vi "DB UI - Search-Load Setup.vi"(8 "error in (no error)":errorcluster, 11 "Refnums":T4) -> (0 "Error Out":errorcluster, 1 "{Cancel}":bool, 2 "Transaction":T3, 3 "1D Results":string[](array[string]))   [LabVIEW 2020]
uses:
  Control/Combo Box.ctl
  Control/DB - Refnums.ctl
  Control/Setup - Part Details - Item Details.ctl
  <vilib>/Utility/miscctls.llb/LVRectTypeDef.ctl
  Control/Transaction Cluster.ctl
  Control/Debug Tab.ctl
  <vilib>/Utility/miscctls.llb/LVRowAndColumnUnsignedTypeDef.ctl
  <vilib>/Utility/miscctls.llb/LVPointTypeDef.ctl
  <vilib>/Utility/miscctls.llb/LVRowAndColumnTypeDef.ctl
  Control/DB - Setup Item Enum.ctl
panel:
  in  "OR [CaptionOnly]":string caption="OR"
  in  "Tab Control":T1
  out "Get Clicked Column Header":i32
  in  "Ascending":bool
  out "Time":u32
  out "x":u32
  out "y":u32
  out "Front Panel Window:Panel Bounds":T2
  out "2D Results":string[][](array[string])=[["Production", "OperationNo1"], ["Production", "Qty1"], ["Production", "NCRNo1"], ["Production", "CustomerID1"], ["Production", "Customer1"], ["Production", "Project1"], ["Production", "SalesOrderNo1"], ["Production", "SalesOrderItemNo1"], ["Production", "MaterialNo1"], ["Production", "MaterialRev1"], ["Production", "MaterialDesc1"], ["Production", "SerialNos1"], ["Production", "UnitOfQty1"]]
  out "Drop Down":bool
  in  "CellBG New Cells":u32(colorbox)=16777225
  in  "CellBG Unused Cells":u32(colorbox)=16777238
  in  "CellBG ColHdrs":u32(colorbox)=11776947
  out "MHandler Error":errorcluster
  in  "Criteria [CaptionOnly]":string caption="Criteria"
  in  "Cancel":bool caption="Report Execute Search"
  in  "Open":bool caption="Report Execute Search"
  in  "Search":bool caption="Report Execute Search"
  in  "Report List":i32(listbox)=-1 caption="List"
  in  "OrderNo":T5 caption="Order No."
  in  "TransactionNo":T5 caption="Transaction No."
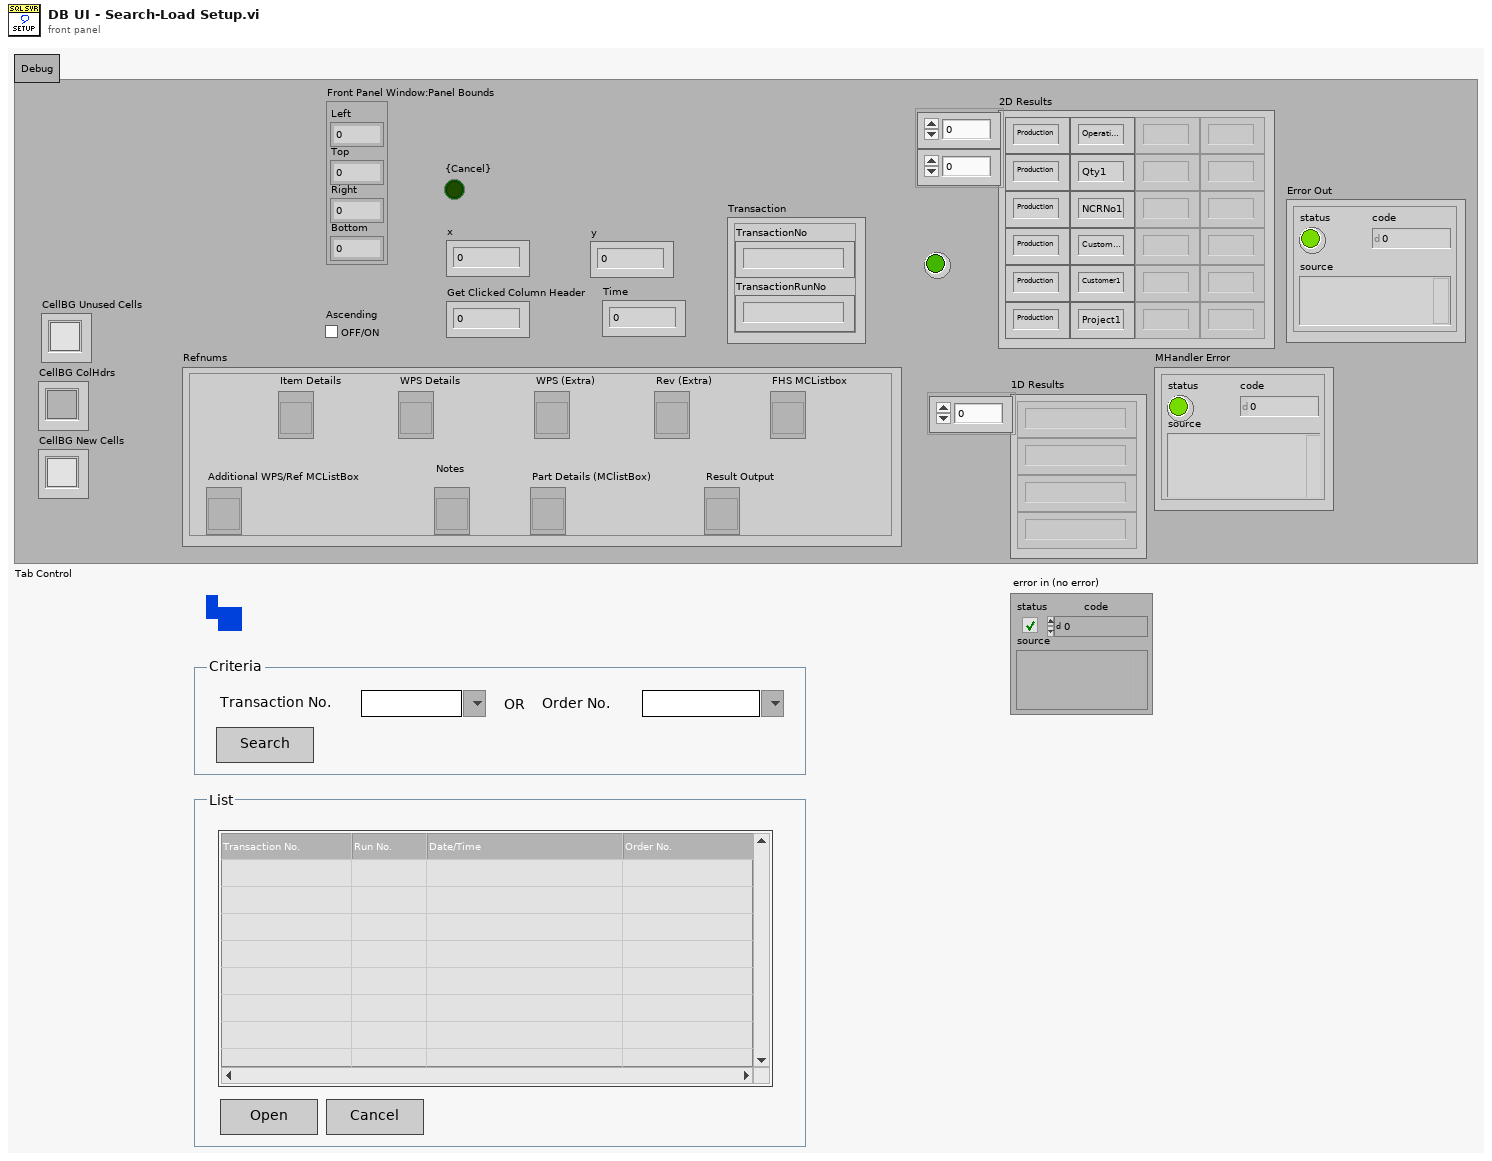
[diagram p1: front panel]
types:
  T1 = typedef "Debug Tab.ctl" = enum32{"Debug"}
  T2 = typedef "LVRectTypeDef.ctl" = cluster{"Left":i16, "Top":i16, "Right":i16, "Bottom":i16}
  T3 = typedef "Transaction Cluster.ctl" = cluster{"TransactionNo":string, "TransactionRunNo":string}
  T4 = typedef "DB - Refnums.ctl" = cluster{"Item Details":refnum<vi>, "WPS Details":refnum<vi>, "WPS (Extra)":refnum<vi>, "Rev (Extra) ":refnum<vi>, "FHS MCListbox":refnum<vi>, "Additional WPS/Ref MCListBox":refnum<vi>, "Notes":refnum<vi>, "Part Details (MClistBox)":refnum<vi>, "Result Output":refnum<vi>}
  T5 = typedef "Combo Box.ctl" = string
  T6 = typedef "LVPointTypeDef.ctl" = cluster{"Horizontal":i16, "Vertical":i16}
  T7 = typedef "LVRowAndColumnUnsignedTypeDef.ctl" = cluster{"Row":u32, "Column":u32}
  T8 = typedef "LVRowAndColumnTypeDef.ctl" = cluster{"Row":i32, "Column":i32}
  T9 = typedef "DB - Setup Item Enum.ctl" = enum16{"SELECT [Plant],[OrderNo]", "INSERT [Setup].[Header]", "INSERT [Setup].[Item]", "INSERT [Setup].[ProcedureItem]", "SELECT [TransactionNo]", "SELECT [TransactionNo], others", "SELECT [OrderNo]", "SELECT [OrderNo], others", "SELECT h.[TransactionNo], i.[OrderNo]", "SELECT [Setup].[ProcedureItem]", "SELECT [EquipmentxId]"}
  T10 = enum8{"Enabled", "Disabled", "Disabled and Grayed Out"}
  T11 = cluster{"TransactionNo":string, "TransactionRunNo":string}
  T12 = typedef "eventvkey.ctl" = enum16{"ASCII", "Enter", "Return", "Shift", "Ctrl", "Alt", "Cmd", "Opt", "Caps", "NumLock", "Clear", "Break", "Up", "Down", "Left", "Right", "Insert", "Delete", "Home", "End", "PageUp", "PageDown", "Escape", "Help", "Pause", "ScrollLock", "F1", "F2", "F3", "F4", "F5", "F6", "F7", "F8", "F9", "F10", "F11", "F12", "F13", "F14", "F15", "F16", "F17", "F18", "F19", "F20", "F21", "F22", "F23", "F24", "Play", "VolumeUp", "VolumeDown", "Mute", "Two Byte Char"}
  T13 = typedef "LVPoint32TypeDef.ctl" = cluster{"Horizontal":i32, "Vertical":i32}
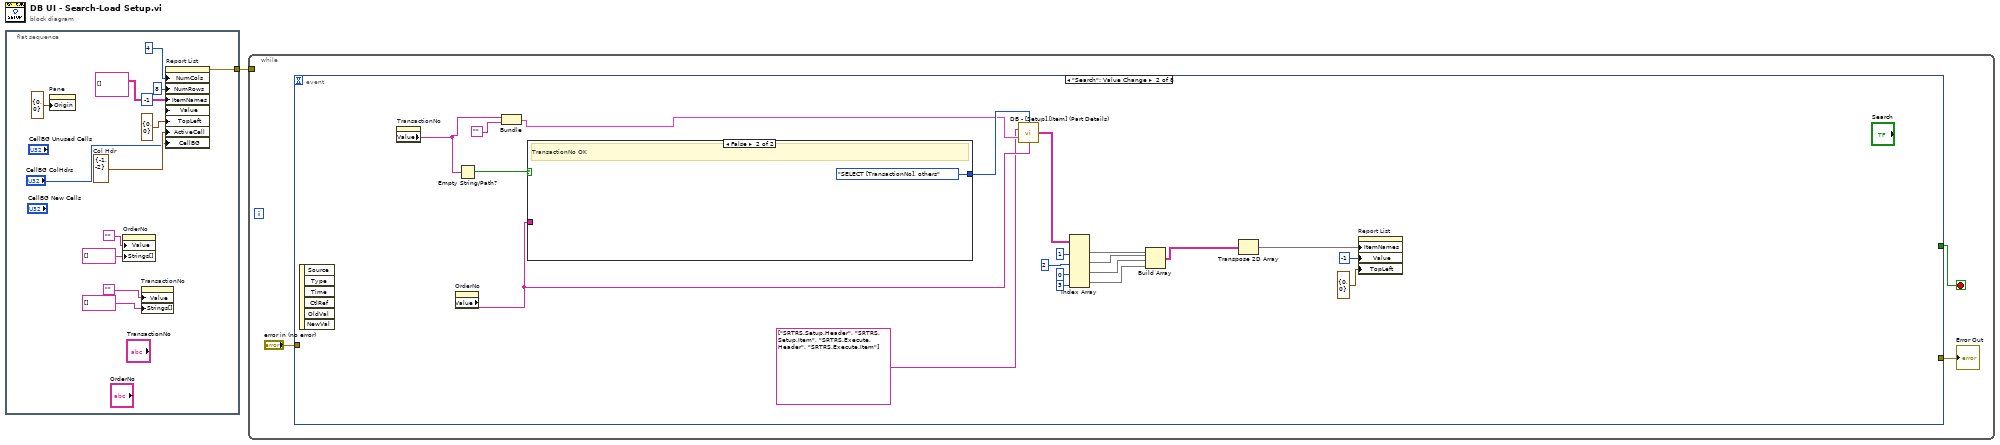
[diagram p0: block diagram]
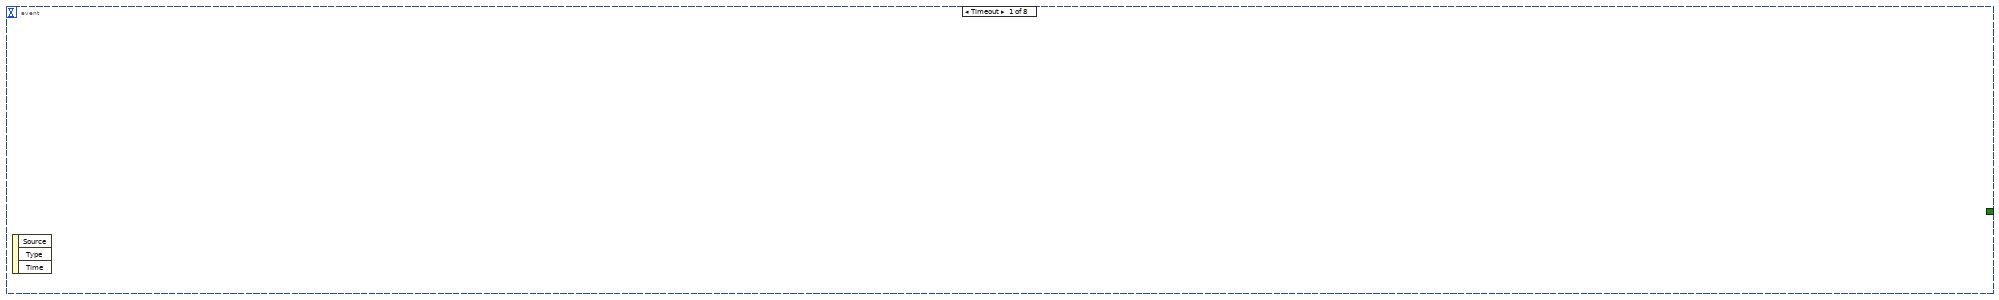
[diagram p2: hidden frame]
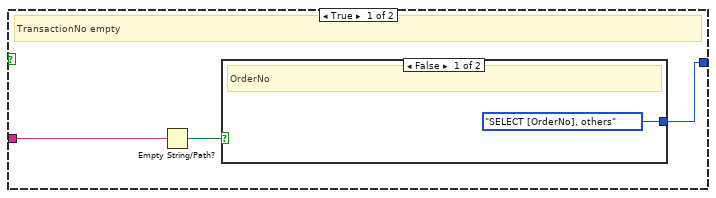
[diagram p3: hidden frame]
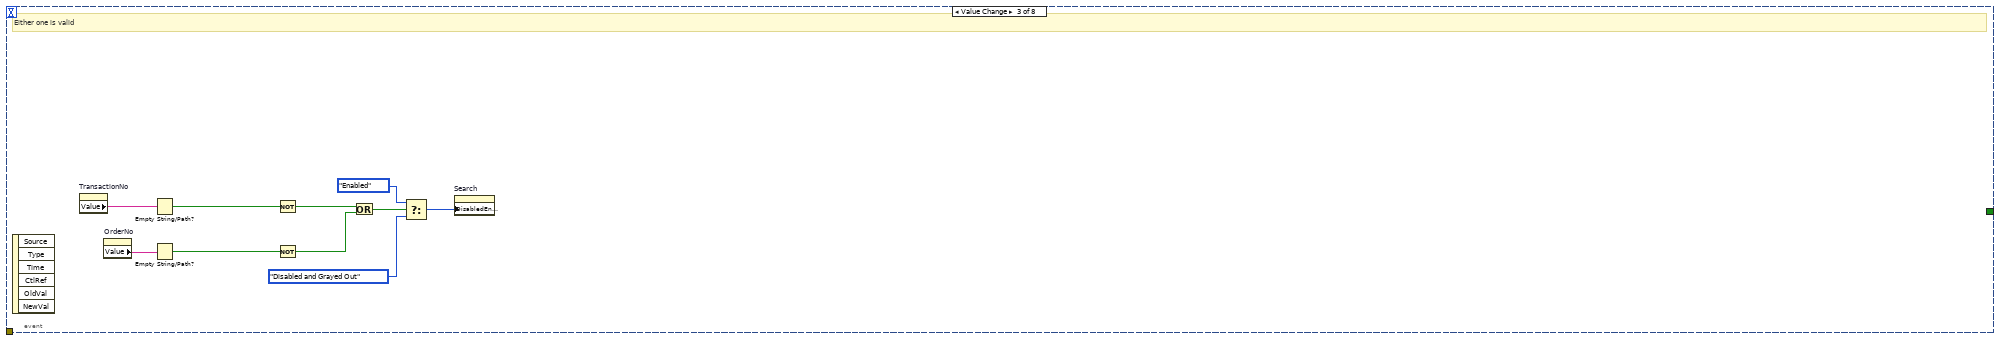
[diagram p5: hidden frame]
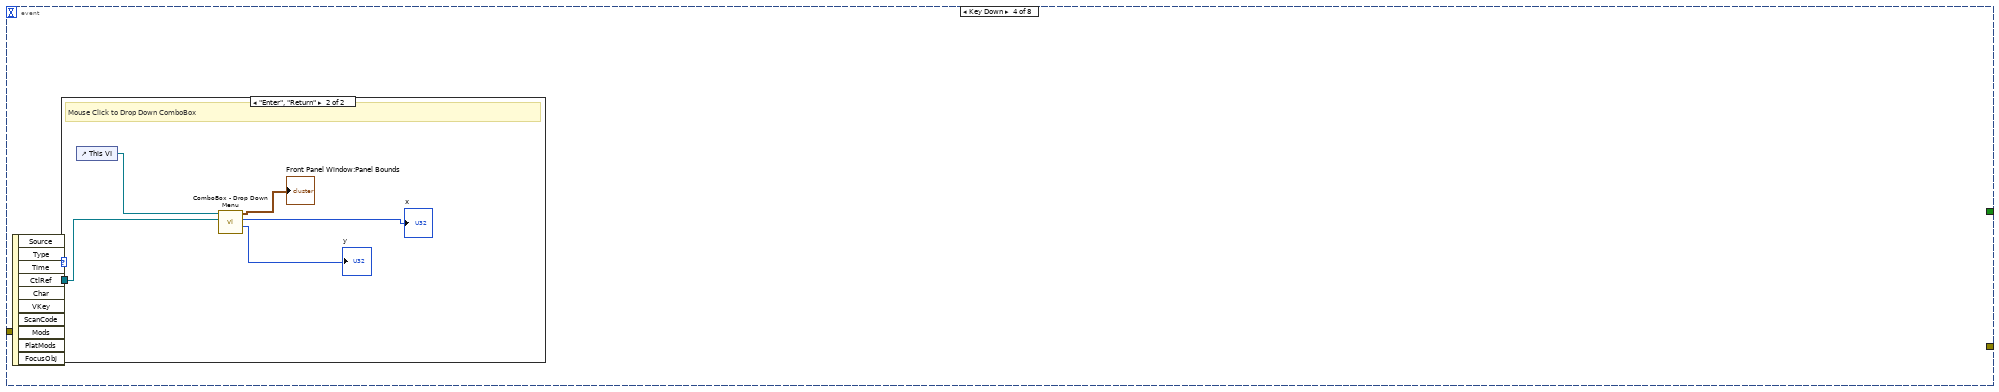
[diagram p6: hidden frame]
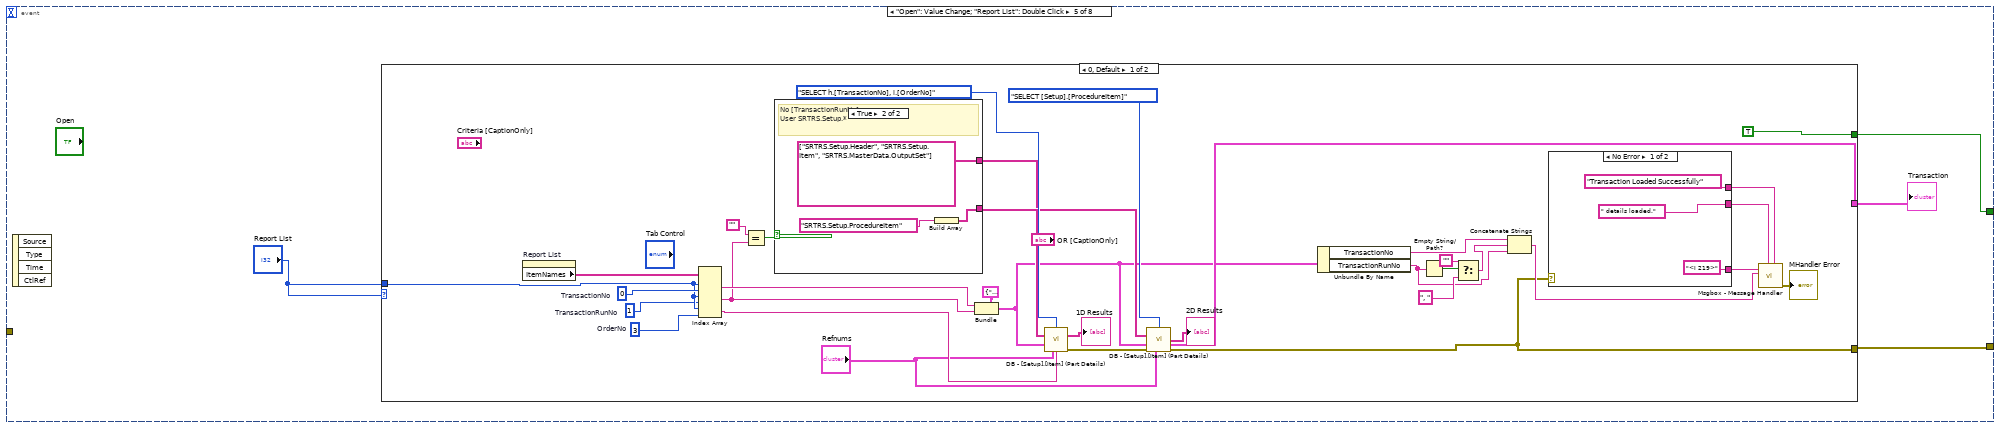
[diagram p8: hidden frame]
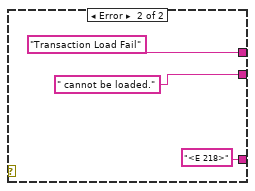
[diagram p9: hidden frame]
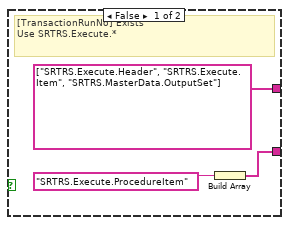
[diagram p10: hidden frame]
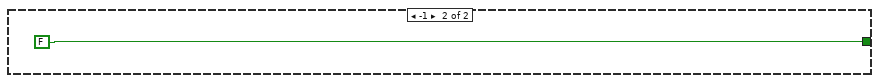
[diagram p11: hidden frame]
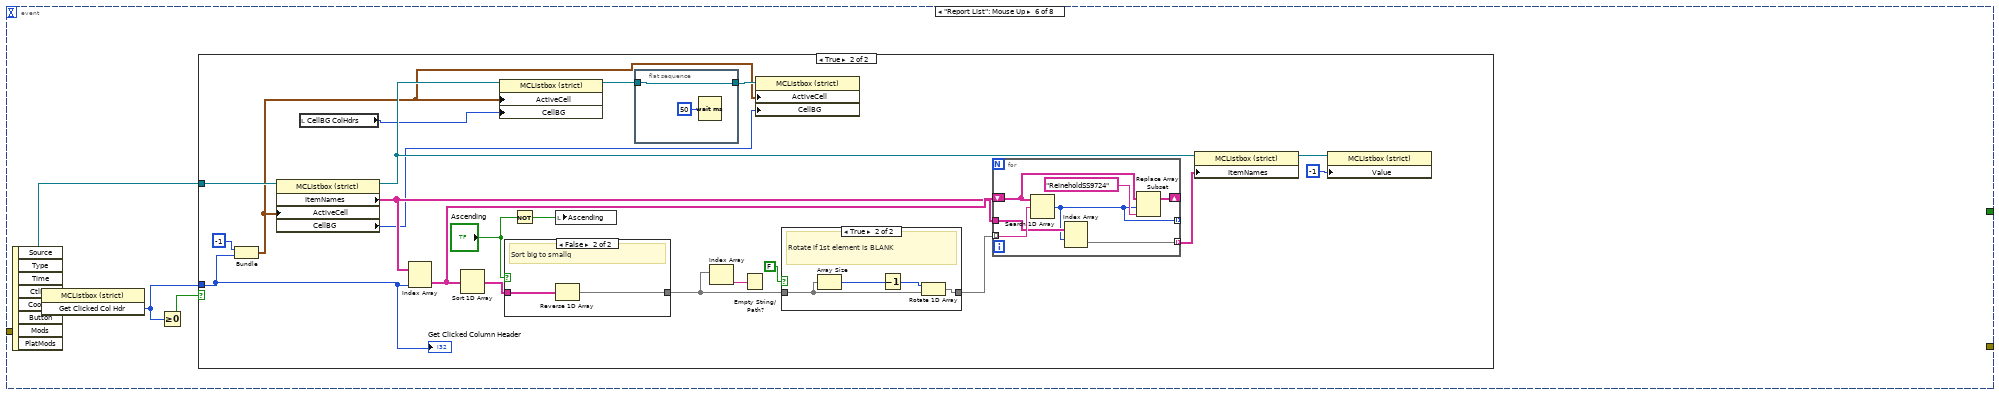
[diagram p12: hidden frame]
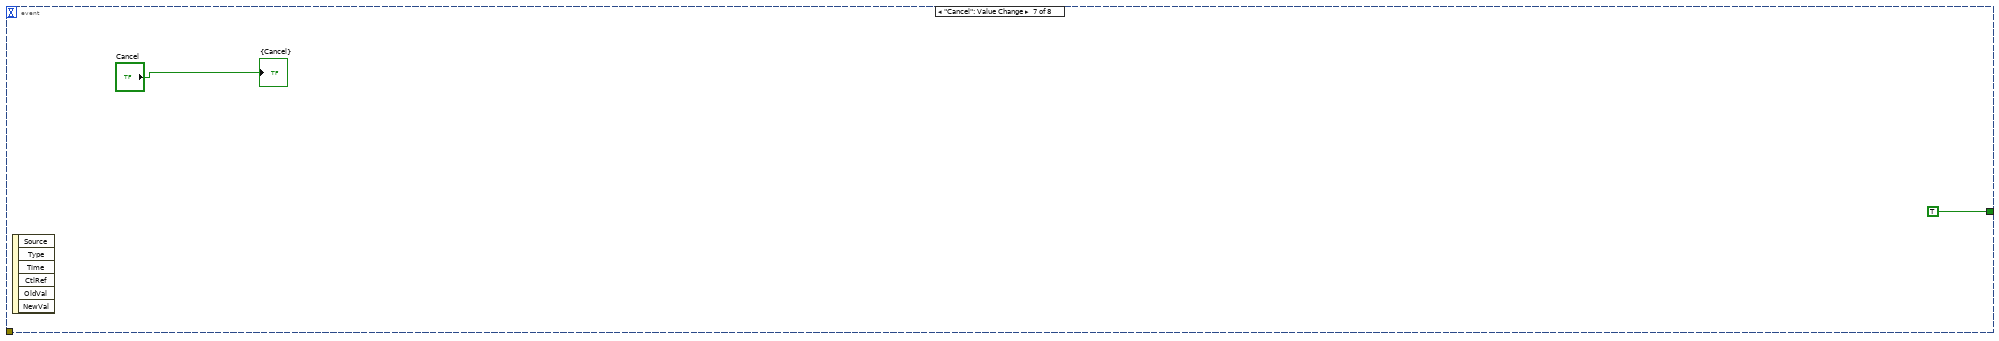
[diagram p16: hidden frame]
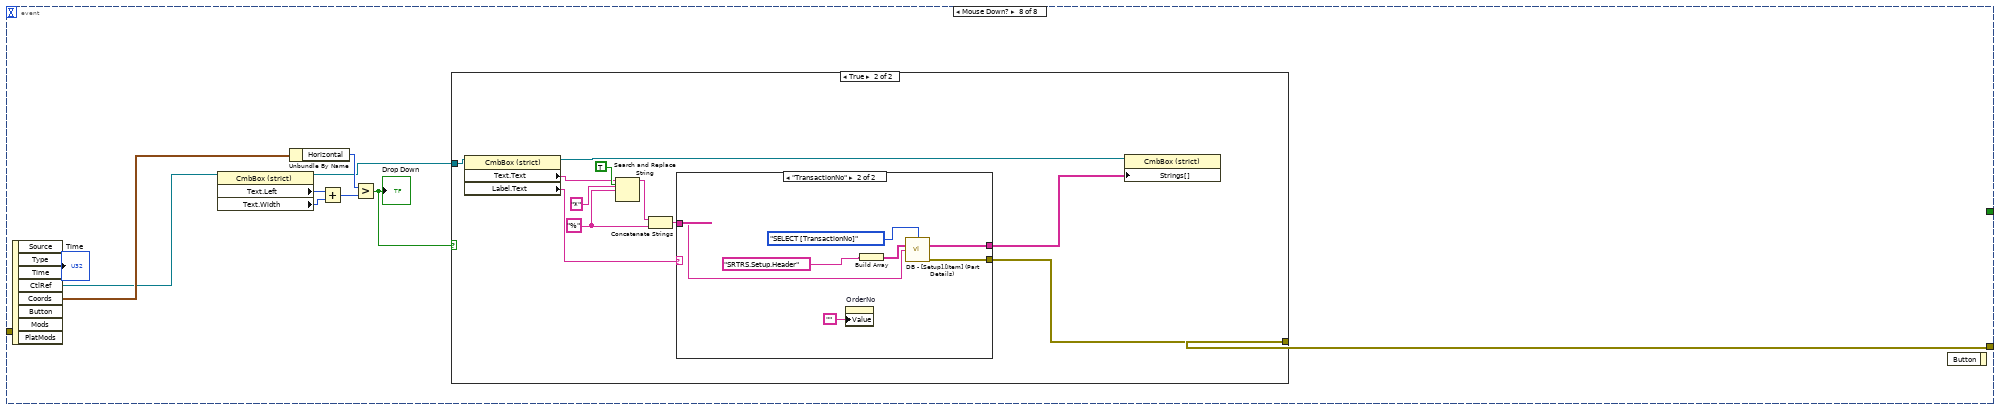
[diagram p17: hidden frame]
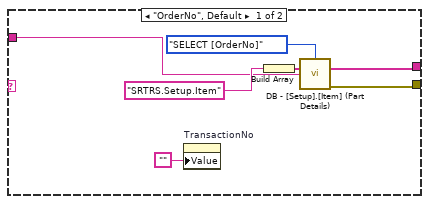
[diagram p19: hidden frame]
diagram:
  n1 = flat-sequence {
    tunnel: [w13] -> w1
    frame #0 {
      w3 = T8 {"Row"=-1, "Column"=-2}  # Col Hdr
      n2 = property on="Pane" class="Pane"("Origin"=T6 {"Horizontal"=0, "Vertical"=0}) -> ()  [unwired: 2 in, 2 out]
      n3 = property on="OrderNo" class="CmbBox (strict)"("Value"="", "Strings[]"=string[] [] ("Strings []")) -> ()  [unwired: 2 in, 2 out]
      n4 = property on="TransactionNo" class="CmbBox (strict)"("Value"="", "Strings[]"=string[] [] ("Strings []")) -> ()  [unwired: 2 in, 2 out]
      n5 = property on="Report List" class="MCListbox (strict)"("NumCols"=u32 4 ("Number of Columns"), "NumRows"=u32 8 ("Number of Rows"), "ItemNames"=string[][] [] ("Item Names"), "Value"=-1 ("Report List"), "TopLeft"=T7 {"Row"=0, "Column"=0} ("Top Left Visible Cell"), "ActiveCell"=w3, "CellBG"="CellBG ColHdrs") -> (error out=w13:errorcluster)  [unwired: 2 in, 1 out]
    }
  }
  n6 = while {
    tunnel: w1 -> [_]
    stop <- w17 stop-if-true
    n7 = event shown="[1] \"Search\": Value Change" {
      selector: _ -> [_ _ _ _ _ _ _ _]
      dyn-events: _ -> [_ _ _ _ _ _ _ _]
      timeout: _ -> [_ _ _ _ _ _ _ _]
      tunnel: [_ _ _ _ w62 _ TRUE ("Cancel") _] -> w17
      tunnel: [_ _ _ _ w60 _ _ w163] -> w16
      tunnel: "error in (no error)" -> [_ _ _ _ _ _ _ _]
      event Timeout {
        n8 = event-data() -> ()  [unwired: 1 in, 3 out]
      }
      event "Search": Value Change {
        n9 = event-data() -> ()  [unwired: 1 in, 6 out]
        n10 = property on="TransactionNo" class="CmbBox (strict)"() -> ("Value"=w21:T5)  [unwired: 2 in, 2 out]
        n11 = property on="OrderNo" class="CmbBox (strict)"() -> ("Value"=w35:T5)  [unwired: 2 in, 2 out]
        n12 = Empty String/Path?(string/path=w21) -> (empty?=w37:bool)
        n13 = Bundle("Value"=w21, "") -> (w20:cluster{"Value":T5, string})  [unwired: 1 in]
        n14 = case shown="False" w37 {
          tunnel: w35 -> [w40 _]
          tunnel: [w38 DB_-_Setup_Item_Enum."SELECT [TransactionNo], others" ("DB - Setup Item Enum")] -> w36
          frame True {
            # "TransactionNo empty"
            n15 = Empty String/Path?(string/path=w40) -> (empty?=w39:bool)
            n16 = case shown="False" w39 {
              tunnel: [DB_-_Setup_Item_Enum."SELECT [OrderNo], others" ("DB - Setup Item Enum") _] -> w38
              frame False {
                # "OrderNo"
              }
              frame True {
                # "OrderNo empty"
              }
            }
          }
          frame False {
            # "TransactionNo OK"
          }
        }
        n17 = call "DB - [Setup].[Item] (Part Details).vi"("DB - Setup Item Enum"=w36, "DB.Schema.Table Array"=string[] ["SRTRS.Setup.Header", "SRTRS.Setup.Item", "SRTRS.Execute.Header", "SRTRS.Execute.Item"], "Transaction"=w20, "OrderNo"=w35) -> ("2D Results"=w32:string[][])  [unwired: 6 in, 5 out]
        n18 = Index Array(array=w32, index (col) #1=1 ("disabled index (col)"), index (col) #2=2 ("index (col)"), index (col) #3=0 ("index (col)"), index (col) #4=3 ("index (col)")) -> (element #1=w30:string[], element #2=w28:string[], element #3=w26:string[], element #4=w25:string[])  [unwired: 4 in]
        n19 = Build Array(w30, w28, w26, w25) -> (w24:string[][])
        n20 = Transpose 2D Array(2D array=w24) -> (transposed array=w23:string[][])
        n21 = property on="Report List" class="MCListbox (strict)"("ItemNames"=w23, "Value"=-1 ("Report List"), "TopLeft"=T7 {"Row"=0, "Column"=0} ("Top Left Visible Cell")) -> ()  [unwired: 2 in, 2 out]
      }
      event Value Change {
        # "Either one is valid"
        n22 = event-data() -> ()  [unwired: 1 in, 6 out]
        n23 = property on="TransactionNo" class="CmbBox (strict)"() -> ("Value"=w52:T5)  [unwired: 2 in, 2 out]
        n24 = property on="OrderNo" class="CmbBox (strict)"() -> ("Value"=w51:T5)  [unwired: 2 in, 2 out]
        n25 = Empty String/Path?(string/path=w52) -> (empty?=w50:bool)
        n26 = Empty String/Path?(string/path=w51) -> (empty?=w49:bool)
        n27 = Not(x=w50) -> (.not. x?=w48:bool)
        n28 = Not(x=w49) -> (.not. x?=w47:bool)
        n29 = Or(x=w48, y=w47) -> (x .or. y?=w46:bool)
        n30 = Select(t=T10."Enabled" ("Disabled"), s=w46, f=T10."Disabled and Grayed Out" ("Disabled")) -> (s? t:f=w44:T10)
        n31 = property on="Search" class="Bool"("DisabledEnum"=w44) -> ()  [unwired: 2 in, 2 out]
      }
      event Key Down {
        n32 = event-data() -> ("CtlRef"=w53:refnum<vi>, "VKey"=w54:T12)  [unwired: 1 in, 8 out]
        n33 = case shown="\"Enter\", \"Return\"" w54 {
          tunnel: w53 -> [_ w58]
          frame "ASCII", Default {
          }
          frame "Enter", "Return" {
            # "Mouse Click to Drop Down ComboBox"
            n34 = control-ref of="This VI"() -> (w59:refnum<vi>)
            n35 = call "ComboBox - Drop Down Menu.vi"("CtlRef"=w58, "VI in (This VI)"=w59) -> ("y"=→"y":u32, "x"=→"x":u32, "Front Panel Window:Panel Bounds"=→"Front Panel Window:Panel Bounds":T2)  [unwired: 7 in]
          }
        }
      }
      event "Open": Value Change; "Report List": Double Click {
        n36 = event-data() -> ()  [unwired: 1 in, 4 out]
        n37 = case shown="0, Default" "Report List" {
          tunnel: "Report List" -> [w87 _]
          tunnel: [w65 _] -> w60
          tunnel: [TRUE ("Cancel") FALSE ("Cancel")] -> w62
          tunnel: [w85 _] -> w61
          frame 0, Default {
            w86 = 1  # TransactionRunNo
            w89 = 3  # OrderNo
            w96 = 0  # TransactionNo
            n38 = property on="Report List" class="MCListbox (strict)"() -> ("ItemNames"=w97:string[][])  [unwired: 2 in, 2 out]
            n39 = Index Array(array=w97, index (row) #1=w87, index (col) #1=w96, index (row) #2=w87, index (col) #2=w86, index (row) #3=w87, index (col) #3=w89) -> (element #1=w90:string, element #2=w84:string, element #3=w88:string)
            n40 = Equal?(x="", y=w84) -> (x = y?=w82:bool)
            n41 = case shown="True" w82 {
              tunnel: [w105 w107] -> w80
              tunnel: [string[] ["SRTRS.Execute.Header", "SRTRS.Execute.Item", "SRTRS.MasterData.OutputSet"] string[] ["SRTRS.Setup.Header", "SRTRS.Setup.Item", "SRTRS.MasterData.OutputSet"]] -> w79
              frame False {
                # "[TransactionRunNo] Exists\nUse SRTRS.Execute.*"
                n42 = Build Array("SRTRS.Execute.ProcedureItem" ("DB.Schema.Table")) -> (w105:string[])
              }
              frame True {
                # "No [TransactionRunNo]\nUser SRTRS.Setup.*"
                n43 = Build Array("SRTRS.Setup.ProcedureItem" ("DB.Schema.Table")) -> (w107:string[])
              }
            }
            n44 = Bundle(cluster=T11 {"TransactionNo"="", "TransactionRunNo"=""} ("output cluster"), "TransactionNo"=w90, "TransactionRunNo"=w84) -> (w64:T11)
            n45 = call "DB - [Setup].[Item] (Part Details).vi"("DB - Setup Item Enum"=DB_-_Setup_Item_Enum."SELECT h.[TransactionNo], i.[OrderNo]", "DB.Schema.Table Array"=w79, "Transaction"=w64, "DB Refnums"="Refnums", "OrderNo"=w88) -> ("1D Results"=→"1D Results":string[], "SUMMARY"=w94:errorcluster)  [unwired: 5 in, 4 out]
            n46 = call "DB - [Setup].[Item] (Part Details).vi"("DB - Setup Item Enum"=DB_-_Setup_Item_Enum."SELECT [Setup].[ProcedureItem]", "DB.Schema.Table Array"=w80, "Transaction"=w64, "error in (no error)"=w94, "DB Refnums"="Refnums") -> ("2D Results"=→"2D Results":string[][], "Transaction"=w85:T3, "SUMMARY"=w65:errorcluster)  [unwired: 5 in, 3 out]
            n47 = Unbundle By Name(w64) -> ("TransactionNo"=w70:string, "TransactionRunNo"=w66:string)
            n48 = Empty String/Path?(string/path=w66) -> (empty?=w71:bool)
            n49 = Select(t="", s=w71, f=", ") -> (s? t:f=w67:string)
            n50 = Concatenate Strings(w70, w67, w66) -> (w73:string)
            n51 = case shown="No Error" w65 {
              tunnel: ["<I 219>" ("<.?....> Message Code") "<E 218>" ("<.?....> Message Code")] -> w76
              tunnel: ["Transaction Loaded Successfully" ("Short Description (When DB Not Available)") "Transaction Load Fail" ("Short Description (When DB Not Available)")] -> w75
              tunnel: [" details loaded." ("Description (When DB Not Available)") " cannot be loaded." ("Description (When DB Not Available)")] -> w74
              frame No Error {
              }
              frame Error {
              }
            }
            n52 = call "Msgbox - Message Handler.vi"("Short Description (When DB Not Available)"=w75, "Description (When DB Not Available)"=w74, "Pre-Description"=w73, "<.?....> Message Code"=w76) -> ("MHandler Error"=→"MHandler Error":errorcluster)  [unwired: 5 in, 2 out]
          }
          frame -1 {
          }
        }
        "Transaction" <- w61
      }
      event "Report List": Mouse Up {
        n53 = event-data() -> ("CtlRef"=w113:refnum<vi>)  [unwired: 1 in, 7 out]
        n54 = invoke class="MCListbox (strict)" method="Get Clicked Col Hdr"(reference=w113) -> ("Get Clicked Column Header"=w112:i32)  [unwired: 2 in, 2 out]
        n55 = Greater Or Equal To 0?(x=w112) -> (x >= 0?=w111:bool)
        n56 = case shown="True" w111 {
          tunnel: w113 -> [_ w127]
          tunnel: w112 -> [_ w120]
          frame False {
          }
          frame True {
            n57 = Bundle(-1, "Get Clicked Column Header"=w120) -> (w117:cluster{i32, "Get Clicked Column Header":i32})  [unwired: 1 in]
            n58 = property class="MCListbox (strict)"(reference=w127, "ActiveCell"=w117) -> (reference out=w122:refnum<vi>, "ItemNames"=w126:string[][], "CellBG"=w116:u32)  [unwired: 1 in, 1 out]
            n59 = local read "CellBG ColHdrs"() -> (w114:u32)
            n60 = Index Array(array=w126, index (col)=w120) -> (element=w130:string[])  [unwired: 1 in]
            n61 = Sort 1D Array(array=w130) -> (sorted array=w133:string[])
            n62 = property class="MCListbox (strict)"(reference=w122, "ActiveCell"=w117, "CellBG"=w114) -> (reference out=w119:refnum<vi>)  [unwired: 1 in, 1 out]
            n63 = case shown="False" "Ascending" {
              tunnel: w133 -> [w142 w144]
              tunnel: [w142 w143] -> w128
              frame True {
                # "Sort small to big p"
              }
              frame False {
                # "Sort big to smallq"
                n64 = Reverse 1D Array(array=w144) -> (reversed array=w143:string[])
              }
            }
            n65 = Not(x="Ascending") -> (.not. x?=w123:bool)
            n66 = local write "Ascending"(w123) -> ()
            n67 = flat-sequence {
              tunnel: w119 -> [w136]
              tunnel: [w136] -> w118
              frame #0 {
                n68 = Wait (ms)(milliseconds to wait=u32 50) -> ()  [unwired: 1 out]
              }
            }
            n69 = Index Array(array=w128) -> (element=w129:string)  [unwired: 1 in]
            n70 = Empty String/Path?(string/path=w129) -> ()  [unwired: 1 out]
            n71 = property class="MCListbox (strict)"(reference=w118, "ActiveCell"=w117, "CellBG"=w116) -> ()  [unwired: 1 in, 2 out]
            n72 = case shown="True" FALSE {
              tunnel: w128 -> [w137 w140]
              tunnel: [w137 w141] -> w125
              frame False {
              }
              frame True {
                # "Rotate if 1st element is BLANK"
                n73 = Array Size(array=w140) -> (size(s)=w139:i32)
                n74 = Decrement(x=w139) -> (x-1=w138:i32)
                n75 = Rotate 1D Array(1:w140, 2:w138) -> (0:w141:string[])
              }
            }
            n76 = for {
              tunnel: w125 -> [w151] mode=indexing
              shift-right: [w148] -> _
              shift-left: w130 -> [w150]
              tunnel: [w145] -> _ mode=indexing
              tunnel: w126 -> [w147]
              tunnel: [w146] -> w134 mode=indexing
              n77 = Search 1D Array(1D array=w150, element=w151) -> (index of element=w145:i32)  [unwired: 1 in]
              n78 = Index Array(array=w147, index (row)=w145) -> (element=w146:string[])  [unwired: 1 in]
              n79 = Replace Array Subset(array=w150, new element="ReineholdSS9724" ("new element/subarray"), index=w145) -> (w148:string[])
            }
            n80 = property class="MCListbox (strict)"(reference=w122, "ItemNames"=w134) -> (reference out=w132:refnum<vi>)  [unwired: 1 in, 1 out]
            n81 = property class="MCListbox (strict)"(reference=w132, "Value"=-1) -> ()  [unwired: 1 in, 2 out]
            "Get Clicked Column Header" <- w120
          }
        }
      }
      event "Cancel": Value Change {
        n82 = event-data() -> ()  [unwired: 1 in, 6 out]
        "{Cancel}" <- "Cancel"
      }
      event Mouse Down? {
        n83 = event-data() -> ("Time"=→"Time":u32, "CtlRef"=w156:refnum<vi>, "Coords"=w159:T13)  [unwired: 1 in, 5 out]
        n84 = property on="Property Node" class="CmbBox (strict)"(reference=w156) -> (reference out=w155:refnum<vi>, "Text.Left"=w161:i32, "Text.Width"=w160:u32)  [unwired: 1 in, 1 out]
        n85 = Unbundle By Name(w159) -> ("Horizontal"=w158:i32)
        n86 = Add(x=w161, y=w160) -> (x+y=w157:u32)
        n87 = Greater?(x=w158, y=w157) -> (0:w154:bool)
        "Drop Down" <- w154
        n88 = case shown="True" w154 {
          tunnel: [_ w174] -> w163
          tunnel: w155 -> [_ w168]
          frame False {
          }
          frame True {
            w169 = "%" ("replace string (\"\")")
            n89 = property on="Property Node" class="CmbBox (strict)"(reference=w168) -> (reference out=w166:refnum<vi>, "Text.Text"=w172:string, "Label.Text"=w164:string)  [unwired: 1 in, 1 out]
            n90 = Search and Replace String(replace all?=TRUE ("replace all? (F)"), input string=w172, search string="*", replace string=w169) -> (result string=w170:string)  [unwired: 4 in, 3 out]
            n91 = Concatenate Strings(w170, w169) -> (w165:string)
            n92 = case shown="\"TransactionNo\"" w164 {
              tunnel: [w178 w188] -> w174
              tunnel: [w180 w186] -> w167
              tunnel: w165 -> [w175 w182]
              frame "OrderNo", Default {
                n93 = property on="TransactionNo" class="CmbBox (strict)"("Value"="") -> ()  [unwired: 2 in, 2 out]
                n94 = Build Array("SRTRS.Setup.Item" ("DB.Schema.Table")) -> (w177:string[])
                n95 = call "DB - [Setup].[Item] (Part Details).vi"("DB - Setup Item Enum"=DB_-_Setup_Item_Enum."SELECT [OrderNo]", "DB.Schema.Table Array"=w177, "Search Parameters"=w175) -> ("1D Results"=w180:string[], "SUMMARY"=w178:errorcluster)  [unwired: 7 in, 4 out]
              }
              frame "TransactionNo" {
                n96 = property on="OrderNo" class="CmbBox (strict)"("Value"="") -> ()  [unwired: 2 in, 2 out]
                n97 = Build Array("SRTRS.Setup.Header" ("DB.Schema.Table")) -> (w184:string[])
                n98 = call "DB - [Setup].[Item] (Part Details).vi"("DB - Setup Item Enum"=DB_-_Setup_Item_Enum."SELECT [TransactionNo]", "DB.Schema.Table Array"=w184, "Search Parameters"=w182) -> ("1D Results"=w186:string[], "SUMMARY"=w188:errorcluster)  [unwired: 7 in, 4 out]
              }
            }
            n99 = property on="Property Node" class="CmbBox (strict)"(reference=w166, "Strings[]"=w167) -> ()  [unwired: 1 in, 2 out]
          }
        }
        n100 = event-data() -> ()  [unwired: 2 in, 1 out]
      }
    }
    "Error Out" <- w16
  }
